vi "Dumb Dashboard Batch Operation.vi"(5 "Operation":enum16{"Save", "Load"}(ring), 7 "Refnum in":T2, 8 "Names List":string[](array[string]), 10 "Section":string, 11 "Named Controls in":T1) -> (2 "Count":i32, 3 "Warnings List":string)   [LabVIEW 2013]
uses:
  <vilib>/Utility/config.llb/Config Data RefNum.ctl
  Named Control.ctl
  <vilib>/Utility/config.llb/NI_LVConfig.lvlib
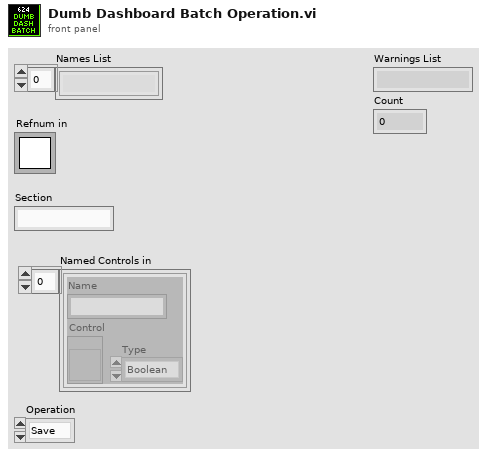
[diagram p1: front panel]
types:
  T1 = typedef "Named Control.ctl" = cluster{"Name":string, "Control":refnum<vi>, "Type":enum16{"Boolean", "Double"}}[]
  T2 = typedef "NI_LVConfig.lvlib/Config Data RefNum.ctl" = refnum<k1>
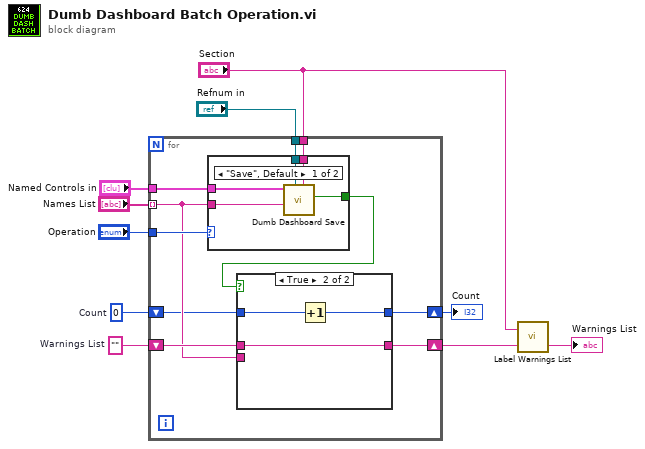
[diagram p0: block diagram]
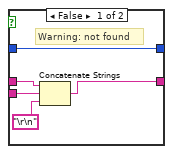
[diagram p2: hidden frame]
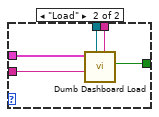
[diagram p3: hidden frame]
diagram:
  w5 = 0  # Count
  w6 = ""  # Warnings List
  n1 = for {
    tunnel: "Names List" -> [w13] mode=indexing
    tunnel: "Named Controls in" -> [w19]
    tunnel: "Operation" -> [w20]
    tunnel: "Refnum in" -> [w18]
    tunnel: "Section" -> [w17]
    shift-right: [w14] -> w3
    shift-left: w6 -> [w15]
    shift-right: [w12] -> w4
    shift-left: w5 -> [w11]
    n2 = case shown="\"Save\", Default" w20 {
      tunnel: w19 -> [w33 w36]
      tunnel: w13 -> [w30 w35]
      tunnel: w18 -> [w32 w38]
      tunnel: w17 -> [w31 w37]
      tunnel: [w29 w34] -> w16
      frame "Save", Default {
        # "Read from control,\nsave to file"
        n3 = call "Dumb Dashboard Save.vi"("section"=w31, "refnum"=w32, "Name"=w30, "Named Controls"=w33) -> ("Found"=w29:bool)  [unwired: 7 in]
      }
      frame "Load" {
        # "Read from file, set control"
        n4 = call "Dumb Dashboard Load.vi"("section"=w37, "refnum"=w38, "Name"=w35, "Named Controls"=w36) -> ("Found"=w34:bool)  [unwired: 7 in]
      }
    }
    n5 = case shown="True" w16 {
      tunnel: w15 -> [w25 w28]
      tunnel: [w24 w28] -> w14
      tunnel: w13 -> [w22 _]
      tunnel: w11 -> [w21 w27]
      tunnel: [w21 w26] -> w12
      frame False {
        # "Warning: not found"
        n6 = Concatenate Strings(w25, w22, "\r\n") -> (w24:string)
      }
      frame True {
        n7 = Increment(x=w27) -> (x+1=w26:i32)
      }
    }
  }
  "Count" <- w4
  n8 = call "Label Warnings List.vi"("Warnings List in"=w3, "Section"="Section") -> ("Warnings List out"=→"Warnings List":string)  [unwired: 1 in]
